vi "Cell Set Source Current.vi"(7 "Box ID":u8, 8 "error in (no error)":errorcluster, 9 "Source Current Limit (mA)":dbl, 10 "Channel":u16, 11 "ENET in":refnum<class "ENET_BS120x.lvclass">) -> (0 "error out":errorcluster, 3 "ENET out":refnum<class "ENET_BS120x.lvclass">)   [LabVIEW 2021, in "BS120x Driver.lvlib" / "ENET_BS120x.lvclass"]
uses:
  ENET_BS120x.lvclass
  BS120x.lvclass
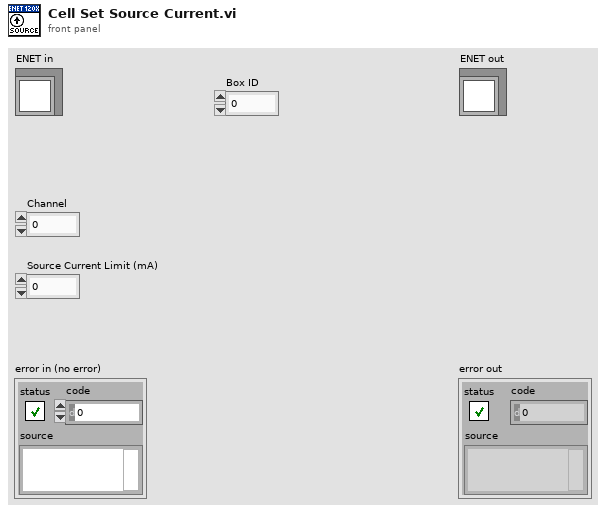
[diagram p1: front panel]
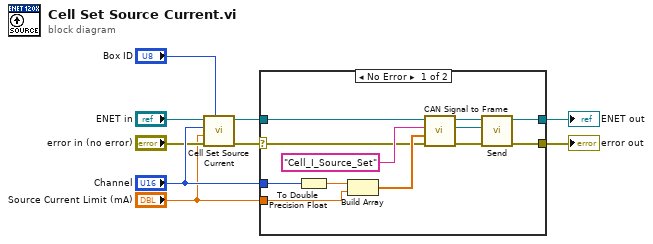
[diagram p0: block diagram]
diagram:
  n1 = call-parent "Cell Set Source Current.vi"("Box ID"="Box ID", "error in (no error)"="error in (no error)", "Source Current Limit (mA)"="Source Current Limit (mA)", "Channel"="Channel", "BS120x in"="ENET in") -> ("error out"=w3:errorcluster, "BS120x out"=w6:refnum<class "ENET_BS120x.lvclass">)  [unwired: 5 in]
  n2 = case shown="No Error" w3 {
    selector: w3 -> [w10 w22]
    tunnel: [w15 w22] -> w9
    tunnel: [w14 w23] -> w8
    tunnel: w6 -> [w13 w23]
    tunnel: "Channel" -> [w12 _]
    tunnel: "Source Current Limit (mA)" -> [w11 _]
    frame No Error {
      n3 = To Double Precision Float(number=w12) -> (double precision float=w21:dbl)
      n4 = Build Array(w21, w11) -> (w20:dbl[])
      n5 = call "CAN Signal to Frame.vi"("error in (no error)"=w10, "Data Array"=w20, "Frame"="Cell_I_Source_Set", "ENET in"=w13) -> ("error out"=w16:errorcluster, "Data"=w17:refnum<class "Data.lvclass">, "ENET out"=w18:refnum<class "ENET_BS120x.lvclass">)  [unwired: 5 in]
      n6 = call "Send.vi"("error in (no error)"=w16, "Data"=w17, "ENET in"=w18) -> ("error out"=w15:errorcluster, "ENET out"=w14:refnum<class "ENET_BS120x.lvclass">)  [unwired: 7 in]
    }
    frame Error {
    }
  }
  "error out" <- w9
  "ENET out" <- w8
